vi "pumpsec_09_8.vi"(0 "reset":i32, 1 "master":i32, 4 "manual":i32, 5 "pause":i32, 7 "Port":i32=10, 8 "pump_type":i32, 9 "port, Reglo D":i32, 14 "Target":dbl[](array[numeric])=[10.0, 2.0, 0.0, 0.0, 0.0, 0.0, 0.0, 0.0, 0.0, 0.0], 16 "fr_manual":dbl, 17 "Time":dbl[](array[numeric])=[4.0, 2.0, 0.0, 0.0, 0.0, 0.0, 0.0, 0.0, 0.0, 0.0]) -> (2 "pumpCtrl":dbl, 3 "totaltarget":dbl, 6 "target_step":dbl, 11 "time_to_target":dbl, 12 "step_fr":dbl, 13 "amount_step":dbl, 15 "Reglo D":dbl, 19 "reset_out":dbl, 20 "Scale":dbl, 21 "mA":dbl format="%#_2g", 23 "elapsed_step":dbl, 24 "Scale actual":dbl, 25 "params":dbl[](array[numeric]), 27 "PAM":dbl)   [LabVIEW 2015]
uses:
  BERTTA.dll
panel:
  out "amount_step_previous":dbl
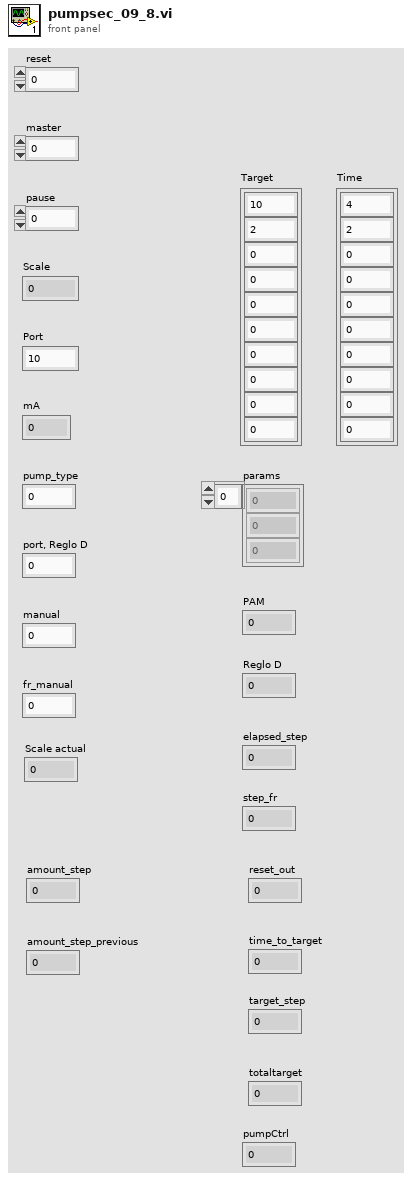
[diagram p1: front panel]
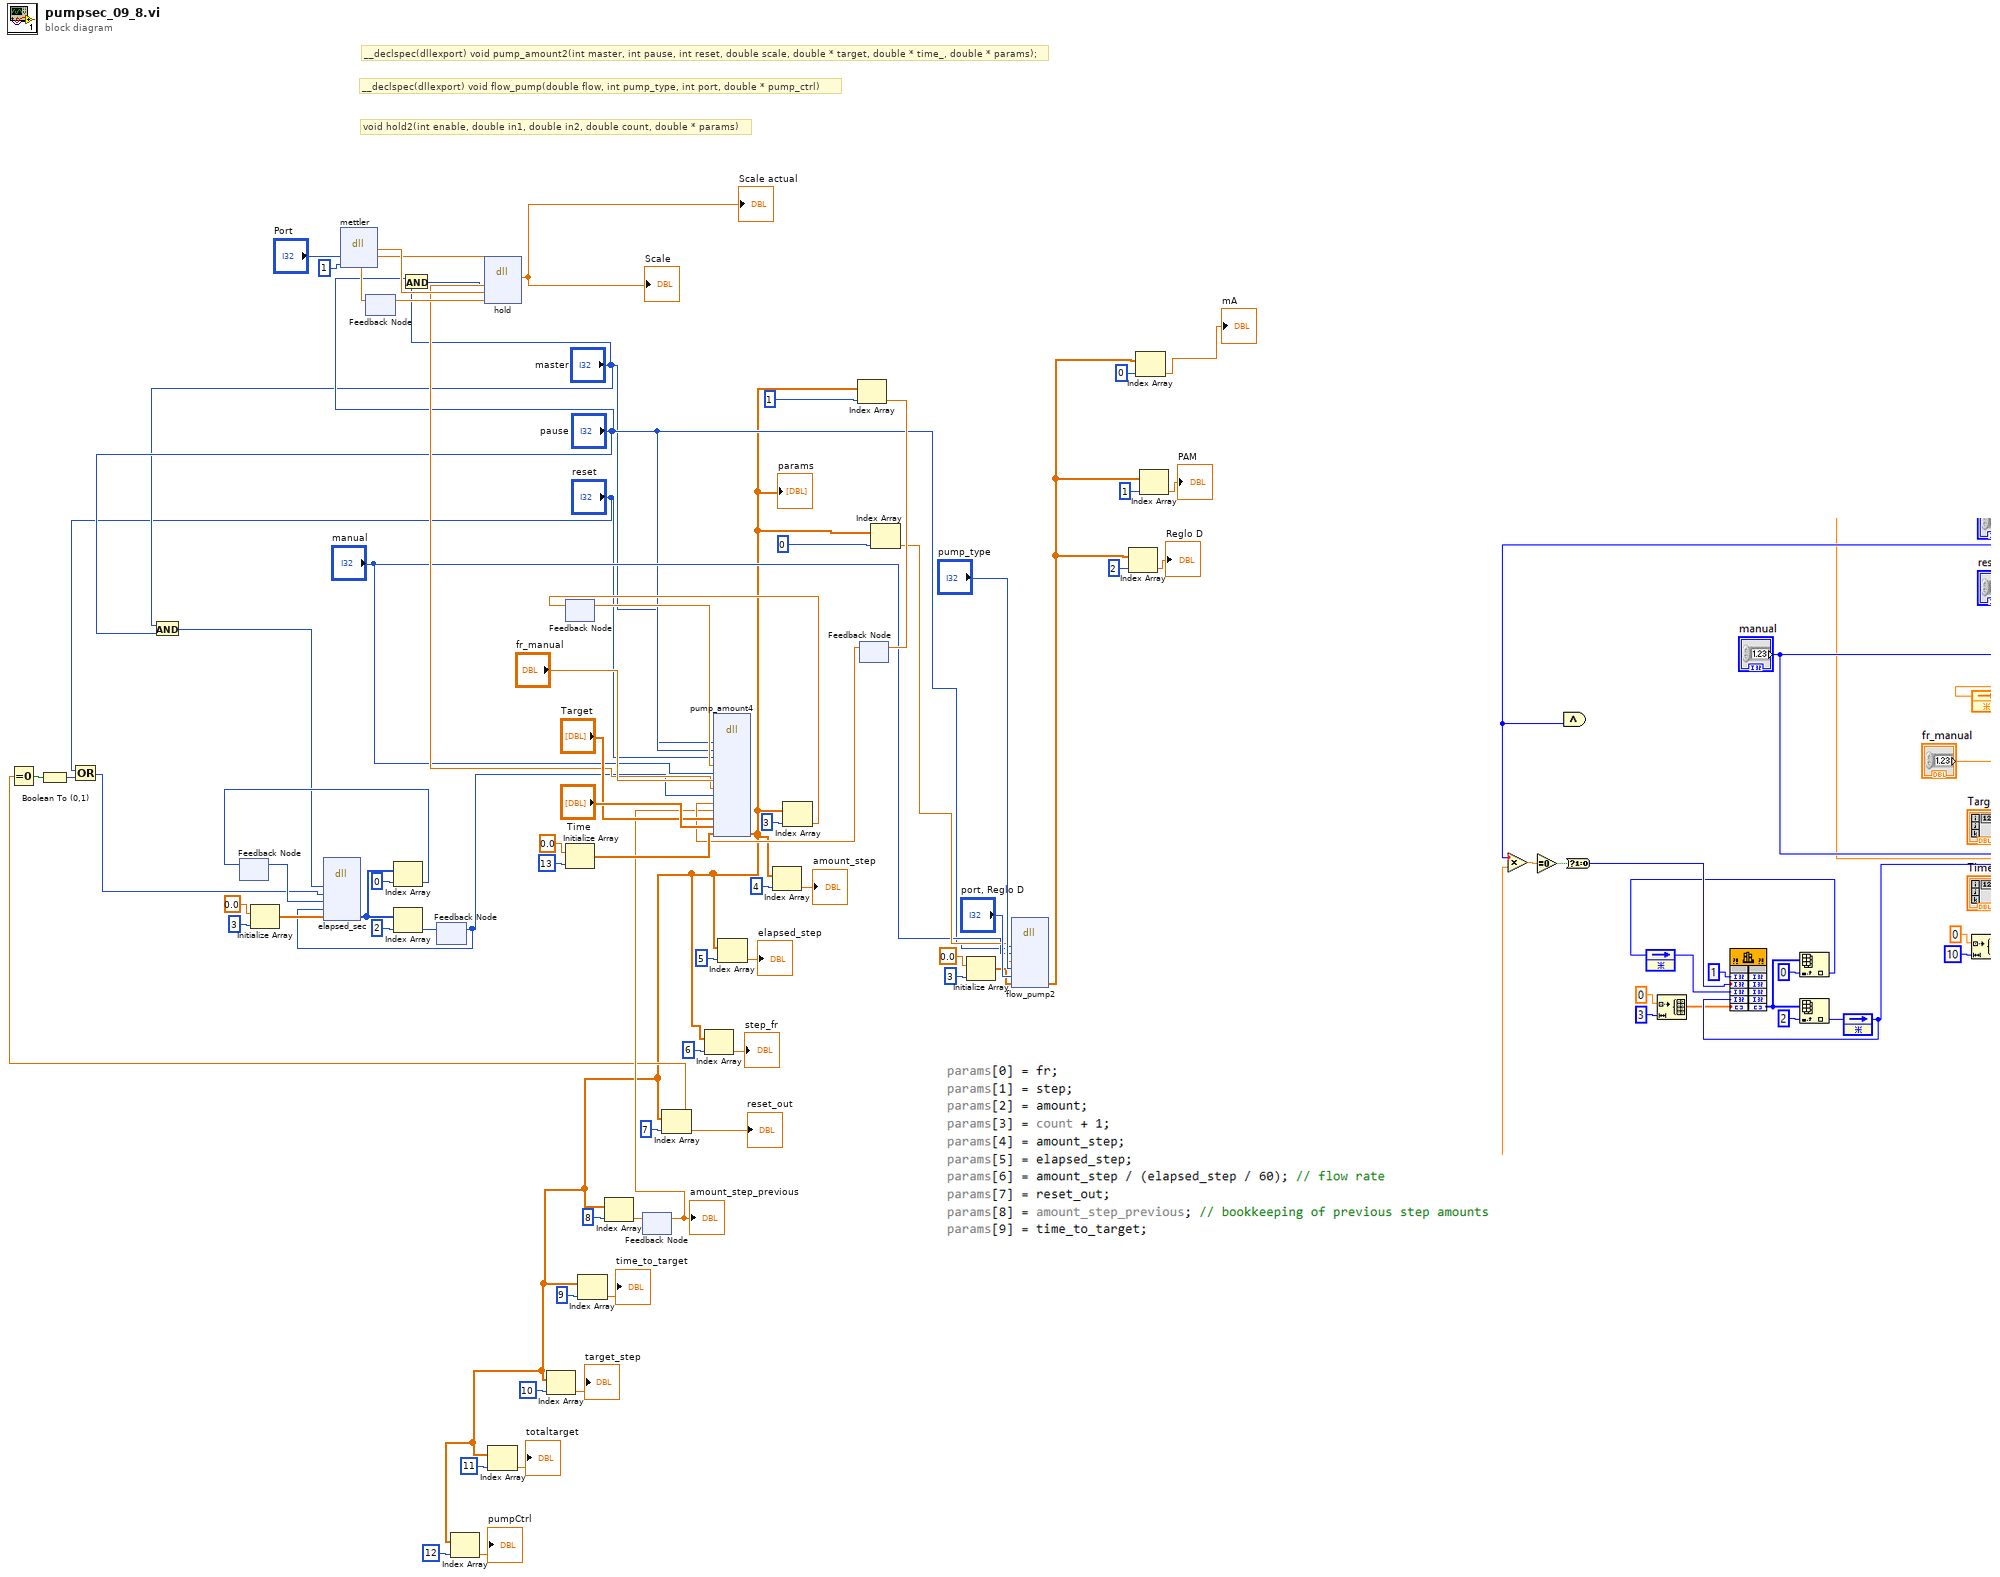
[diagram p0: block diagram]
diagram:
  # "void hold2(int enable, double in1, double in2, double count, double * params)"
  # "__declspec(dllexport) void flow_pump(double flow, int pump_type, int port, double * pump_ctrl)"
  # "__declspec(dllexport) void pump_amount2(int master, int pause, int reset, double scale, double * target, double * time_, double * params);"
  n1 = And(x="master", y="pause") -> (x .and. y?=w13:i32)
  n2 = feedback #1() -> (w25:i32)  [unwired: 1 in]
  n3 = Initialize Array(0.0 ("element"), 3 ("dimension size")) -> (w29:dbl[])
  n4 = dll-call lib="C:/Users/shresplab/OneDrive - Kemira Oyj/Documents/Visual Studio 2017/Projects/Bertta/BERTTA/x64/Debug/BERTTA.dll" fn="mettler"("port"="Port", "msg"=1) -> ("return type"=w49:dbl)  [unwired: 5 in, 2 out]
  n5 = feedback #2() -> (w48:dbl)  [unwired: 1 in]
  n6 = And(x="pause", y="master") -> (x .and. y?=w46:i32)
  n7 = feedback #3() -> (w23:i32)  [unwired: 1 in]
  n8 = dll-call lib="C:/Users/shresplab/OneDrive - Kemira Oyj/Documents/Visual Studio 2017/Projects/Bertta/BERTTA/x64/Debug/BERTTA.dll" fn="hold"("enable"=w46, "in1"=w49, "in2"=w48) -> ("return type"=w47:dbl)  [unwired: 6 in, 2 out]
  "Scale" <- w47
  "Scale actual" <- w47
  n9 = feedback-in #2(w47) -> ()
  n10 = feedback #4() -> (w43:dbl)  [unwired: 1 in]
  n11 = Initialize Array(0.0 ("element"), 13 ("dimension size")) -> (w56:dbl[])
  n12 = feedback #5() -> (w20:dbl)  [unwired: 1 in]
  "amount_step_previous" <- w20
  n13 = feedback #6() -> (w33:dbl)  [unwired: 1 in]
  n14 = dll-call lib="C:/Users/shresplab/OneDrive - Kemira Oyj/Documents/Visual Studio 2017/Projects/Bertta/BERTTA/x64/Debug/BERTTA.dll" fn="pump_amount4"("master"="master", "pause"="pause", "reset"="reset", "count"=w43, "manual"="manual", "fr_manual"="fr_manual", "scale"=w47, "elapsed"=w23, "step_previous"=w33, "amount_step_previous"=w20, "target"="Target", "time_"="Time", "params"=w56) -> ("params"=w1:dbl[])  [unwired: 16 in, 2 out]
  "params" <- w1
  n15 = Index Array(array=w1, index=12) -> (element=→"pumpCtrl":dbl)
  n16 = Index Array(array=w1, index=11) -> (element=→"totaltarget":dbl)
  n17 = Index Array(array=w1, index=10) -> (element=→"target_step":dbl)
  n18 = Index Array(array=w1, index=9) -> (element=→"time_to_target":dbl)
  n19 = Index Array(array=w1, index=8) -> (element=w21:dbl)
  n20 = feedback-in #5(w21) -> ()
  n21 = Index Array(array=w1, index=7) -> (element=w10:dbl)
  "reset_out" <- w10
  n22 = Equal To 0?(x=w10) -> (x = 0?=w9:bool)
  n23 = Boolean To (0,1)(Boolean=w9) -> (0, 1=w8:i16)
  n24 = Or(x="reset", y=w8) -> (x .or. y?=w12:i32)
  n25 = dll-call lib="C:/Users/shresplab/OneDrive - Kemira Oyj/Documents/Visual Studio 2017/Projects/Bertta/BERTTA/x64/Debug/BERTTA.dll" fn="elapsed_sec"("enable"=w13, "reset"=w12, "last_time"=w25, "elapsed_last"=w23, "params"=w29) -> ("params"=w27:i32[])  [unwired: 8 in, 2 out]
  n26 = Index Array(array=w27, index=0) -> (element=w26:i32)
  n27 = feedback-in #1(w26) -> ()
  n28 = Index Array(array=w27, index=2) -> (element=w24:i32)
  n29 = feedback-in #3(w24) -> ()
  n30 = Index Array(array=w1, index=6) -> (element=→"step_fr":dbl)
  n31 = Index Array(array=w1, index=5) -> (element=→"elapsed_step":dbl)
  n32 = Index Array(array=w1, index=4) -> (element=→"amount_step":dbl)
  n33 = Index Array(array=w1, index=3) -> (element=w44:dbl)
  n34 = feedback-in #4(w44) -> ()
  n35 = Index Array(array=w1, index=1) -> (element=w34:dbl)
  n36 = feedback-in #6(w34) -> ()
  n37 = Index Array(array=w1, index=0) -> (element=w19:dbl)
  n38 = Initialize Array(0.0 ("element"), 3 ("dimension size")) -> (w61:dbl[])
  n39 = dll-call lib="C:/Users/shresplab/OneDrive - Kemira Oyj/Documents/Visual Studio 2017/Projects/Bertta/BERTTA/x64/Debug/BERTTA.dll" fn="flow_pump2"("enable"="pause", "manual"="manual", "flow"=w19, "pump_type"="pump_type", "port"="port, Reglo D", "pump_ctrl"=w61) -> ("pump_ctrl"=w52:dbl[])  [unwired: 9 in, 2 out]
  n40 = Index Array(array=w52, index=2) -> (element=→"Reglo D":dbl)
  n41 = Index Array(array=w52, index=0) -> (element=→"mA":dbl)
  n42 = Index Array(array=w52, index=1) -> (element=→"PAM":dbl)
